vi "Mode Scan Engine.vi"() -> ()   [LabVIEW 2014]
uses:
  Controls/Standard Action.ctl
  Controls/Standard_Counter_Action.ctl
  <vilib>/Analysis/6fits.llb/Curve Fitting Criteria.ctl
  <vilib>/Analysis/baseanly.llb/Mean (DBL).vi
  <vilib>/Analysis/NI_AALBase.lvlib
  <vilib>/Analysis/NI_AALPro.lvlib
  <vilib>/gmath/NI_Gmath.lvlib
panel:
  in  "Initial Guess":T1={"Amp"=7.0, "Center"=7.0, "Sigma"=7.0, "Offset"=7.0}
  in  "Manual Initial Guess":bool
  in  "Upper Limit":dbl=7.0
  in  "Lower Limit":dbl=7.0
  out "Metric":cluster{dbl[], dbl[]}[](graph)
  out "Image":sgl[][](graph)
  in  "Step Size (nm)":u16=7
  in  "Number of Steps":u16=7
  in  "Get Image":bool
  in  "Scan Next Mode":bool
  in  "Metric":u16(ring) items=["Max Intensity", "No Zero Mean", "Threshold Mean"]
  in  "Fit Type":u16(ring) items=["Guassian", "Quadratic"]
  in  "Mode":i32(ring) items=["1", "2", "3", "4", "5", "6", "7", "8", "9", "10", "11", "12", "13", "14", "15", "16", "17", "18", "19", "20", "21", "22", "23", "24", "25", "26", "27", "28", "29", "30", "31", "32", "33", "34", "35", "36", "37", "38", "39", "40", "41", "42", "43", "44", "45", "46", "47", "48", "49", "50", "51", "52", "53", "54", "55", "56", "57", "58", "59", "60", "61", "62", "63", "64", "65", "66", "67", "68", "69", "70", "71", "72", "73", "74", "75", "76", "77", "78", "79", "80", "81", "82", "83", "84", "85", "86", "87", "88", "89", "90", "91", "92", "93", "94", "95", "96", "97", "98", "99", "100", "101", "102", "103", "104", "105", "106", "107", "108", "109", "110", "111", "112", "113", "114", "115", "116", "117", "118", "119", "120", "121", "122", "123", "124", "125", "126", "127", "128", "129", "130", "131", "132", "133", "134", "135", "136", "137", "138", "139", "140"]
  in  "Apply":bool
  in  "Fit Data":bool
  in  "Scan Mode":bool
  in  "Exit":bool
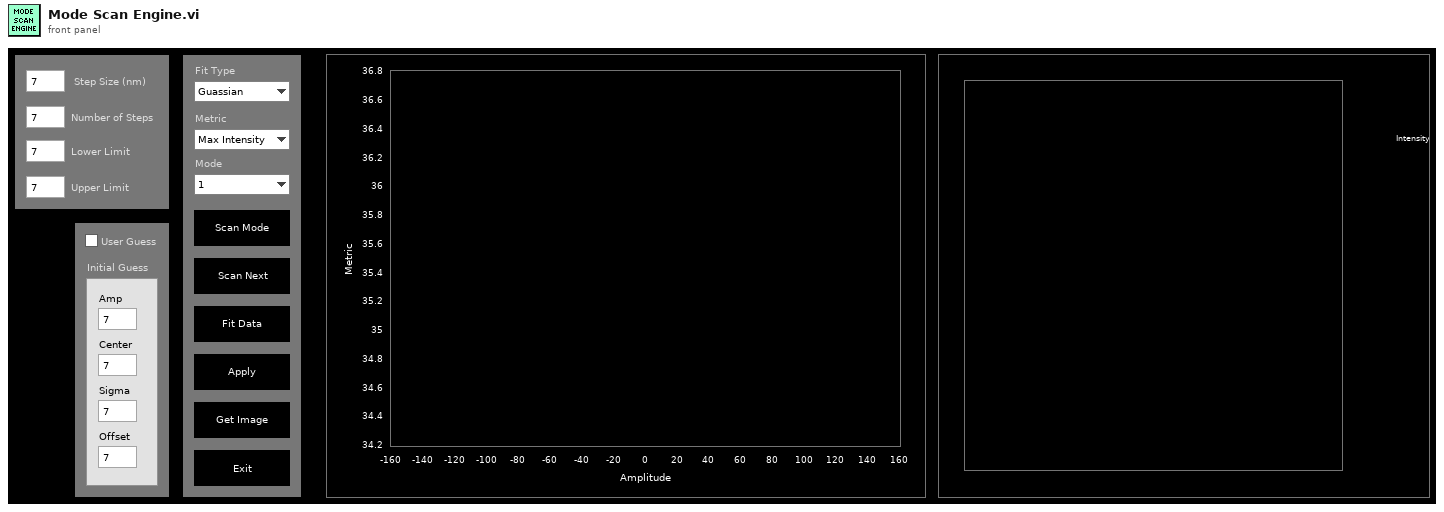
[diagram p1: front panel]
types:
  T1 = cluster{"Amp":dbl, "Center":dbl, "Sigma":dbl, "Offset":dbl}
  T2 = typedef "Standard Action.ctl" = enum16{"Read", "Write"}
  T3 = typedef "MirrorModes.ctl" = cluster{"Mode":string, "Amplitude":dbl}[]
  T4 = typedef "Standard_Counter_Action.ctl" = enum16{"Initialize", "Update Count", "Get Count"}
  T5 = cluster{"amp min":dbl, "amp max":dbl, "center min":dbl, "center max":dbl, "deviation min":dbl, "deviation max":dbl, "offset min":dbl, "offset max":dbl}
  T6 = enum16{"Linear", "Polynomial", "Exponential", "Power"}
  T7 = cluster{"Amplitude Out":dbl[], "Metric Out":dbl[]}
  T8 = cluster{"Amp":dbl, "Numeric":dbl, "Sigma":dbl, "Offset":dbl}
  T9 = typedef "NI_AALPro.lvlib/Curve Fitting Criteria.ctl" = u16
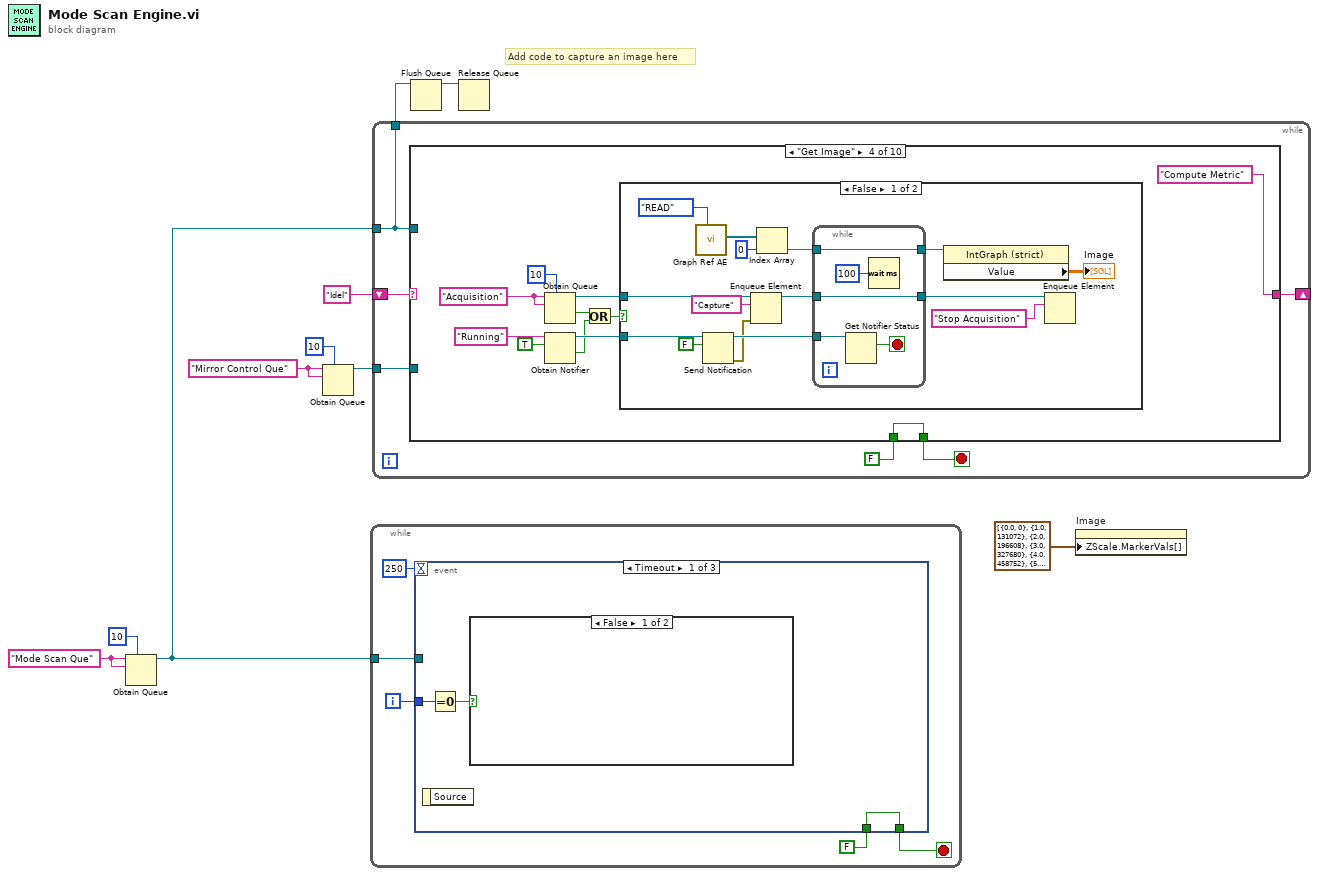
[diagram p0: block diagram]
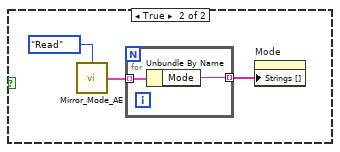
[diagram p2: hidden frame]
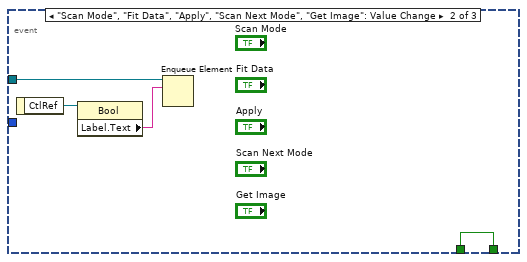
[diagram p3: hidden frame]
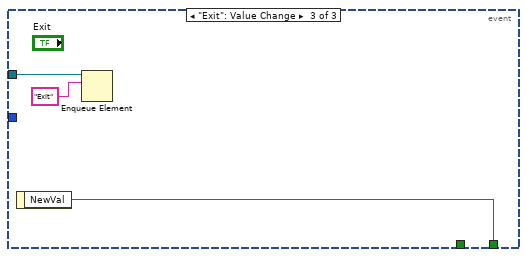
[diagram p4: hidden frame]
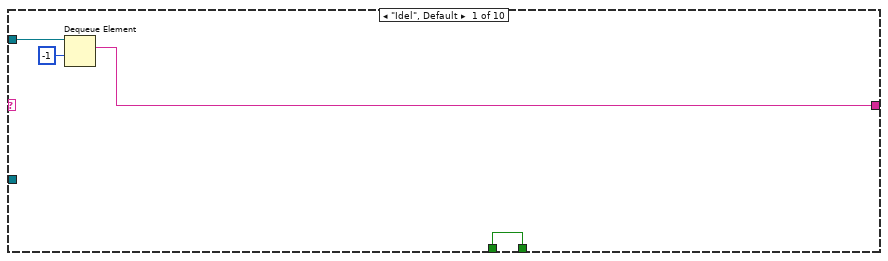
[diagram p5: hidden frame]
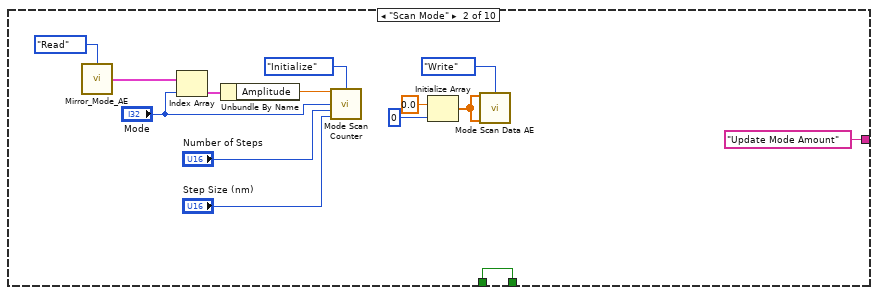
[diagram p6: hidden frame]
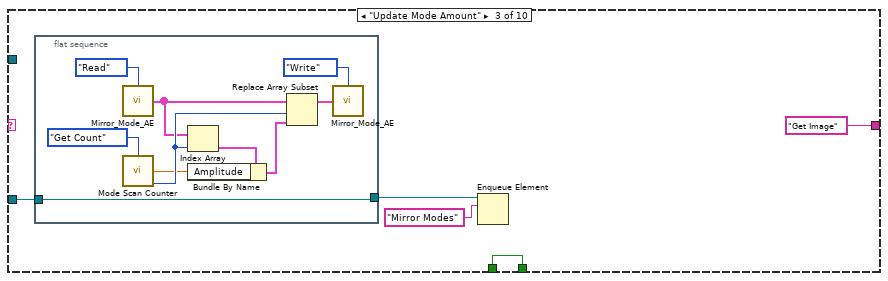
[diagram p7: hidden frame]
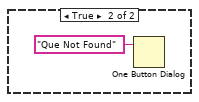
[diagram p8: hidden frame]
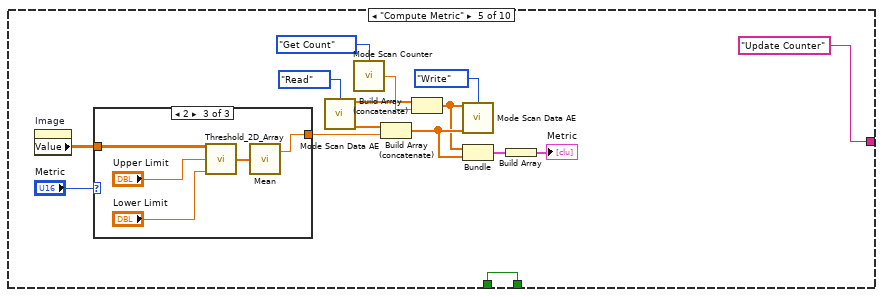
[diagram p9: hidden frame]
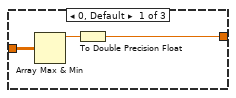
[diagram p10: hidden frame]
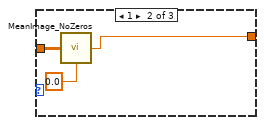
[diagram p11: hidden frame]
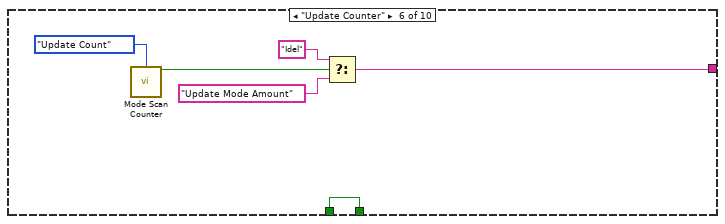
[diagram p12: hidden frame]
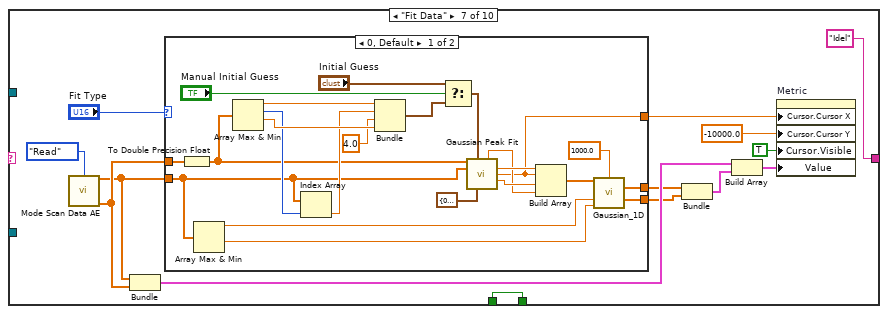
[diagram p13: hidden frame]
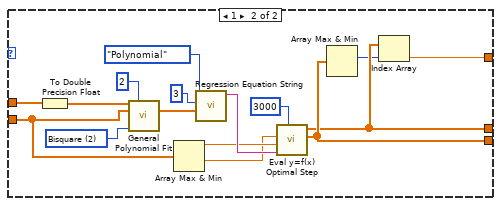
[diagram p14: hidden frame]
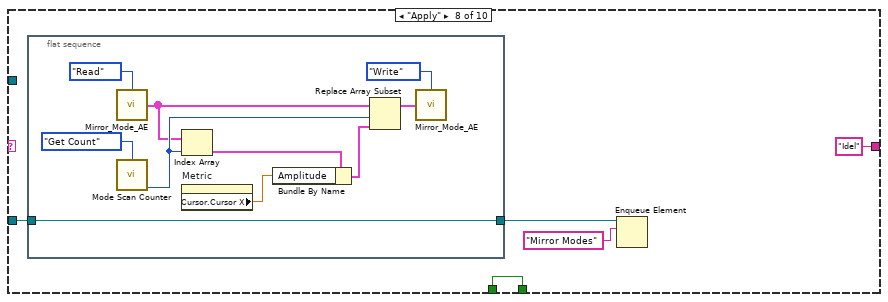
[diagram p15: hidden frame]
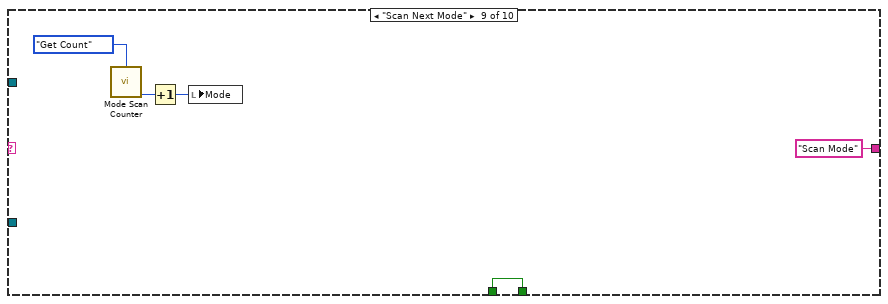
[diagram p16: hidden frame]
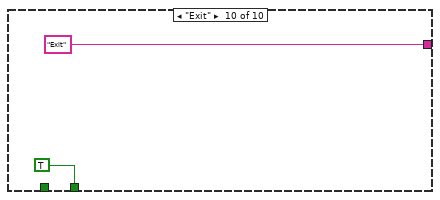
[diagram p17: hidden frame]
diagram:
  w4 = "Mirror Control Que" ("name (unnamed)")
  w9 = "Mode Scan Que" ("name (unnamed)")
  # "Add code to capture an image here"
  n1 = Obtain Queue(max queue size (-1, unlimited)=10, name (unnamed)=w9, element data type=w9) -> (queue out=w7:refnum<queue>)  [unwired: 2 in, 2 out]
  n2 = Obtain Queue(max queue size (-1, unlimited)=10, name (unnamed)=w4, element data type=w4) -> (queue out=w2:refnum<queue>)  [unwired: 2 in, 2 out]
  n3 = while {
    tunnel: w7 -> [w15]
    i -> [w12]
    stop <- w14 stop-if-true
    n4 = event shown="[0] Timeout" {
      selector: _ -> [_ _ _]
      dyn-events: _ -> [_ _ _]
      timeout: 250 -> [_ _ _]
      tunnel: w15 -> [_ w26 w30]
      tunnel: [w18 w24 w28] -> w14
      tunnel: FALSE -> [w18 w24 _]
      tunnel: w12 -> [w17 _ _]
      event Timeout {
        n5 = event-data() -> ()  [unwired: 1 in, 1 out]
        n6 = Equal To 0?(x=w17) -> (x = 0?=w16:bool)
        n7 = case shown="False" w16 {
          frame False {
          }
          frame True {
            n8 = call "Mirror_Mode_AE.vi"("Action"=Standard_Action."Read") -> ("Mirror Modes Out"=w20:T3)  [unwired: 14 in]
            n9 = for {
              tunnel: w20 -> [w23] mode=indexing
              tunnel: [w22] -> w21 mode=indexing
              n10 = Unbundle By Name(w23) -> ("Mode"=w22:string)
            }
            n11 = property on="Mode" class="Ring (strict)"("Strings []"=w21) -> ()  [unwired: 2 in, 2 out]
          }
        }
      }
      event "Scan Mode", "Fit Data", "Apply", "Scan Next Mode", "Get Image": Value Change {
        n12 = event-data() -> ("CtlRef"=w25:refnum<vi>)  [unwired: 1 in]
        n13 = property class="Bool"(reference=w25) -> ("Label.Text"=w27:string)  [unwired: 1 in, 2 out]
        n14 = Enqueue Element(queue=w26, element=w27) -> ()  [unwired: 2 in, 3 out]
      }
      event "Exit": Value Change {
        n15 = event-data() -> ("NewVal"=w28:bool)  [unwired: 1 in]
        n16 = Enqueue Element(queue=w30, element="Exit") -> ()  [unwired: 2 in, 3 out]
      }
    }
  }
  n17 = while {
    shift-right: [w33] -> _
    shift-left: "Idel" -> [w36]
    tunnel: w7 -> [w32]
    tunnel: [w32] -> w6
    tunnel: w2 -> [w31]
    stop <- w35 stop-if-true
    n18 = case shown="\"Get Image\"" w36 {
      tunnel: [w40 w54 w59 w80 w115 w133 w147 w191 w206 TRUE] -> w35
      tunnel: FALSE -> [w40 w54 w59 w80 w115 w133 w147 w191 w206 _]
      tunnel: w32 -> [w38 _ _ _ _ _ _ _ _ _]
      tunnel: [w37 "Update Mode Amount" ("name (unnamed)") "Get Image" ("name (unnamed)") "Compute Metric" ("name (unnamed)") "Update Counter" ("name (unnamed)") w130 "Idel" ("name (unnamed)") "Idel" ("name (unnamed)") "Scan Mode" ("name (unnamed)") "Exit" ("name (unnamed)")] -> w33
      tunnel: w31 -> [_ _ w58 _ _ _ _ w189 _ _]
      frame "Idel", Default {
        n19 = Dequeue Element(queue=w38, timeout in ms (-1)=-1) -> (element=w37:string)  [unwired: 1 in, 3 out]
      }
      frame "Scan Mode" {
        n20 = call "Mirror_Mode_AE.vi"("Action"=Standard_Action."Read") -> ("Mirror Modes Out"=w49:T3)  [unwired: 14 in]
        n21 = Index Array(array=w49, index="Mode") -> (element=w50:cluster{"Mode":string, "Amplitude":dbl})
        n22 = Unbundle By Name(w50) -> ("Amplitude"=w51:dbl)
        n23 = call "Mode Scan Counter.vi"("Center Value"=w51, "Action"=Standard_Counter_Action."Initialize", "Mode"="Mode", "Number of Steps"="Number of Steps", "Step Size"="Step Size (nm)") -> ()  [unwired: 8 in, 3 out]
        n24 = Initialize Array(0.0 ("element"), 0 ("dimension size")) -> (w41:dbl[])
        n25 = call "Mode Scan Data AE.vi"("Amplitude"=w41, "Action"=Standard_Action."Write", "Metric"=w41) -> ()  [unwired: 11 in, 2 out]
      }
      frame "Update Mode Amount" {
        n26 = flat-sequence {
          tunnel: w58 -> [w60]
          tunnel: [w60] -> w56
          frame #0 {
            n27 = call "Mirror_Mode_AE.vi"("Action"=Standard_Action."Read") -> ("Mirror Modes Out"=w63:T3)  [unwired: 14 in]
            n28 = call "Mode Scan Counter.vi"("Action"=Standard_Counter_Action."Get Count") -> ("Output"=w67:dbl, "Current Mode"=w68:i32)  [unwired: 12 in, 1 out]
            n29 = Index Array(array=w63, index=w68) -> (element=w66:cluster{"Mode":string, "Amplitude":dbl})
            n30 = Bundle By Name(cluster=w66, "Amplitude"=w67) -> (w69:cluster{"Mode":string, "Amplitude":dbl})
            n31 = Replace Array Subset(array=w63, new element=w69, index=w68) -> (w65:T3)
            n32 = call "Mirror_Mode_AE.vi"("Action"=Standard_Action."Write", "Mirror Modes In"=w65) -> ()  [unwired: 13 in, 1 out]
          }
        }
        n33 = Enqueue Element(queue=w56, element="Mirror Modes" ("name (unnamed)")) -> ()  [unwired: 2 in, 3 out]
      }
      frame "Get Image" {
        w75 = "Acquisition" ("name (unnamed)")
        n34 = Obtain Queue(max queue size (-1, unlimited)=10, name (unnamed)=w75, element data type=w75) -> (queue out=w78:refnum<queue>, created new?=w72:bool)  [unwired: 2 in, 1 out]
        n35 = Obtain Notifier(name (unnamed)="Running", notification data type=TRUE) -> (notifier out=w77:refnum<notifier>, created new?=w71:bool)  [unwired: 2 in, 1 out]
        n36 = Or(x=w72, y=w71) -> (x .or. y?=w70:bool)
        n37 = case shown="False" w70 {
          tunnel: w78 -> [w84 _]
          tunnel: w77 -> [w82 _]
          frame False {
            n38 = call "Graph Ref AE.vi"("Action"=enum16{"READ", "WRITE"}."READ") -> ("Graph Ref Out"=w92:refnum<vi>[])  [unwired: 10 in]
            n39 = Send Notification(notification=FALSE, notifier=w82) -> (notifier out=w87:refnum<notifier>, error out=w86:errorcluster)  [unwired: 1 in]
            n40 = Enqueue Element(queue=w84, element="Capture", error in (no error)=w86) -> (queue out=w88:refnum<queue>)  [unwired: 1 in, 2 out]
            n41 = Index Array(array=w92, index=0) -> (element=w94:refnum<vi>)
            n42 = while {
              tunnel: w87 -> [w100]
              tunnel: [w98] -> w89
              tunnel: w88 -> [w98]
              tunnel: [w97] -> w95
              tunnel: w94 -> [w97]
              stop <- w99 stop-if-true
              n43 = Get Notifier Status(notifier=w100) -> (current notification=w99:bool)  [unwired: 1 in, 4 out]
              n44 = Wait (ms)(milliseconds to wait=u32 100) -> ()  [unwired: 1 out]
            }
            n45 = property class="IntGraph (strict)"(reference=w95) -> ("Value"=→"Image":sgl[][])  [unwired: 1 in, 2 out]
            n46 = Enqueue Element(queue=w89, element="Stop Acquisition" ("f")) -> ()  [unwired: 2 in, 3 out]
          }
          frame True {
            n47 = One Button Dialog(message="Que Not Found") -> ()  [unwired: 1 in, 1 out]
          }
        }
      }
      frame "Compute Metric" {
        n48 = property on="Image" class="IntGraph (strict)"() -> ("Value"=w102:sgl[][])  [unwired: 2 in, 2 out]
        n49 = case shown="2" "Metric" {
          tunnel: w102 -> [w119 w122 w127]
          tunnel: [w117 w121 w125] -> w109
          frame 0, Default {
            n50 = Array Max & Min(array=w119) -> (max value=w118:sgl)  [unwired: 3 out]
            n51 = To Double Precision Float(number=w118) -> (double precision float=w117:dbl)
          }
          frame 1 {
            n52 = call "MeanImage_NoZeros.vi"("Image IN"=w122, "STDev Factor"=0.0) -> ("No Zero Mean"=w121:dbl)  [unwired: 13 in]
          }
          frame 2 {
            n53 = call "Threshold_2D_Array.vi"("2D Array IN"=w127, "Upper Limit"="Upper Limit", "Lower Limit"="Lower Limit") -> ("Threshold Array Out"=w126:dbl[])  [unwired: 12 in]
            n54 = call-poly <vilib>:"Mean.vi"("X"=w126) -> ("mean"=w125:dbl)  [unwired: 1 out]
          }
        }
        n55 = call "Mode Scan Data AE.vi"("Action"=Standard_Action."Read") -> ("Amplitude Out"=w106:dbl[], "Metric Out"=w107:dbl[])  [unwired: 13 in]
        n56 = call "Mode Scan Counter.vi"("Action"=Standard_Counter_Action."Get Count") -> ("Output"=w108:dbl)  [unwired: 12 in, 2 out]
        n57 = Build Array (concatenate)(w107, w109) -> (w112:dbl[])
        n58 = Build Array (concatenate)(w106, w108) -> (w111:dbl[])
        n59 = call "Mode Scan Data AE.vi"("Amplitude"=w111, "Action"=Standard_Action."Write", "Metric"=w112) -> ()  [unwired: 11 in, 2 out]
        n60 = Bundle(w111, w112) -> (w113:cluster{dbl[], dbl[]})  [unwired: 1 in]
        n61 = Build Array(w113) -> (→"Metric":cluster{dbl[], dbl[]}[])
      }
      frame "Update Counter" {
        n62 = call "Mode Scan Counter.vi"("Action"=Standard_Counter_Action."Update Count") -> ("Scan Done?"=w128:bool)  [unwired: 12 in, 2 out]
        n63 = Select(t="Idel", s=w128, f="Update Mode Amount") -> (s? t:f=w130:string)
      }
      frame "Fit Data" {
        n64 = call "Mode Scan Data AE.vi"("Action"=Standard_Action."Read") -> ("Amplitude Out"=w142:dbl[], "Metric Out"=w143:dbl[])  [unwired: 13 in]
        n65 = Bundle("Amplitude Out"=w142, "Metric Out"=w143) -> (w141:T7)  [unwired: 1 in]
        n66 = case shown="0, Default" "Fit Type" {
          tunnel: w142 -> [w163 w176]
          tunnel: w143 -> [w170 w175]
          tunnel: [w151 w172] -> w136
          tunnel: [w150 w173] -> w139
          tunnel: [w149 w174] -> w138
          frame 0, Default {
            n67 = To Double Precision Float(number=w170) -> (double precision float=w164:dbl[])
            n68 = Array Max & Min(array=w163) -> (max value=w152:dbl, min value=w153:dbl)  [unwired: 2 out]
            n69 = Array Max & Min(array=w164) -> (max value=w169:dbl, max index (indices)=w166:i32, min value=w168:dbl)  [unwired: 1 out]
            n70 = Index Array(array=w163, index=w166) -> (element=w165:dbl)
            n71 = Bundle(w169, "Numeric"=w165, 4.0, w168) -> (w162:cluster{dbl, "Numeric":dbl, dbl, dbl})  [unwired: 1 in]
            n72 = Select(t="Initial Guess", s="Manual Initial Guess", f=w162) -> (s? t:f=w161:T8)
            n73 = call <vilib>:"Gaussian Peak Fit.vi"("Y"=w164, "initial guess"=w161, "X"=w163, "parameter bounds"=T5 {"amp min"=0.0, "amp max"=100000.0, "center min"=-100.0, "center max"=100.0, "deviation min"=0.0, "deviation max"=1000.0, "offset min"=0.0, "offset max"=1000.0}) -> ("offset"=w156:dbl, "amplitude"=w158:dbl, "center"=w151:dbl, "standard deviation"=w157:dbl)  [unwired: 5 in, 3 out]
            n74 = Build Array(w158, w151, w157, w156) -> (w155:dbl[])
            n75 = call "Gaussian_1D.vi"("Parameters In"=w155, "Number of Points"=1000.0, "Max X Value"=w152, "Min X Value"=w153) -> ("X Values"=w150:dbl[], "Y Values"=w149:dbl[])  [unwired: 10 in]
          }
          frame 1 {
            w185 = T9 2 items=["Least Square", "Least Absolute Residual", "Bisquare"] ("method")
            n76 = To Double Precision Float(number=w175) -> (double precision float=w186:dbl[])
            n77 = call <vilib>:"General Polynomial Fit.vi"("Y"=w186, "polynomial order"=2, "X"=w176, "method"=w185) -> ("Polynomial Coefficients"=w182:dbl[])  [unwired: 8 in, 3 out]
            n78 = Array Max & Min(array=w176) -> (max value=w178:dbl, min value=w177:dbl)  [unwired: 2 out]
            n79 = call "Regression Equation String.vi"("coefficients"=w182, "precision"=3, "fit type"=T6."Polynomial") -> ("Formula"=w180:string)  [unwired: 8 in]
            n80 = call <vilib>:"Eval y=f(x) Optimal Step.vi"("number of points"=u32 3000, "formula"=w180, "end"=w178, "start"=w177) -> ("Y Values"=w174:dbl[], "X Values"=w173:dbl[])  [unwired: 1 in, 2 out]
            n81 = Array Max & Min(array=w174) -> (max index (indices)=w171:i32)  [unwired: 3 out]
            n82 = Index Array(array=w173, index=w171) -> (element=w172:dbl)
          }
        }
        n83 = Bundle("X Values"=w139, "Y Values"=w138) -> (w137:cluster{"X Values":dbl[], "Y Values":dbl[]})  [unwired: 1 in]
        n84 = Build Array(w141, w137) -> (w140:cluster{"X Values":dbl[], "Y Values":dbl[]}[])
        n85 = property on="Metric" class="XYGraph (strict)"("Cursor.Cursor X"=w136, "Cursor.Cursor Y"=-10000.0 ("Cursor.Cursor Position:Cursor X"), "Cursor.Visible"=TRUE, "Value"=w140) -> ()  [unwired: 2 in, 2 out]
      }
      frame "Apply" {
        n86 = flat-sequence {
          tunnel: [w193] -> w187
          tunnel: w189 -> [w193]
          frame #0 {
            n87 = call "Mirror_Mode_AE.vi"("Action"=Standard_Action."Read") -> ("Mirror Modes Out"=w196:T3)  [unwired: 14 in]
            n88 = call "Mode Scan Counter.vi"("Action"=Standard_Counter_Action."Get Count") -> ("Current Mode"=w200:i32)  [unwired: 12 in, 2 out]
            n89 = Index Array(array=w196, index=w200) -> (element=w199:cluster{"Mode":string, "Amplitude":dbl})
            n90 = property on="Metric" class="XYGraph (strict)"() -> ("Cursor.Cursor X"=w192:dbl)  [unwired: 2 in, 2 out]
            n91 = Bundle By Name(cluster=w199, "Amplitude"=w192) -> (w201:cluster{"Mode":string, "Amplitude":dbl})
            n92 = Replace Array Subset(array=w196, new element=w201, index=w200) -> (w198:T3)
            n93 = call "Mirror_Mode_AE.vi"("Action"=Standard_Action."Write", "Mirror Modes In"=w198) -> ()  [unwired: 13 in, 1 out]
          }
        }
        n94 = Enqueue Element(queue=w187, element="Mirror Modes" ("name (unnamed)")) -> ()  [unwired: 2 in, 3 out]
      }
      frame "Scan Next Mode" {
        n95 = call "Mode Scan Counter.vi"("Action"=Standard_Counter_Action."Get Count") -> ("Current Mode"=w203:i32)  [unwired: 12 in, 2 out]
        n96 = Increment(x=w203) -> (x+1=w204:i32)
        n97 = local write "Mode"(w204) -> ()
      }
      frame "Exit" {
      }
    }
  }
  n98 = Flush Queue(queue=w6) -> (queue out=w5:refnum<queue>)  [unwired: 1 in, 2 out]
  n99 = Release Queue(queue=w5) -> ()  [unwired: 2 in, 3 out]
  n100 = property on="Image" class="IntGraph (strict)"("ZScale.MarkerVals[]"=cluster{dbl, u32}[] [{0.0, 0}, {1.0, 131072}, {2.0, 196608}, {3.0, 327680}, {4.0, 458752}, {5.0, 589824}, {6.0, 720896}, {7.0, 851971}, {8.0, 983043}, {9.0, 1114115}, {10.0, 1245187}, {11.0, 1376259}, {12.0, 1507331}, {13.0, 1638403}, {14.0, 1769475}, {15.0, 1769479}, {16.0, 2031623}, {17.0, 2162695}, {18.0, 2293767}, {19.0, 2424839}, {20.0, 2555911}, {21.0, 2686983}, {22.0, 2818055}, {23.0, 2949127}, {24.0, 3080203}, {25.0, 3211275}, {26.0, 3342347}, {27.0, 3473419}, {28.0, 3604491}, {29.0, 3735563}, {30.0, 3866635}, {31.0, 3867403}, {32.0, 4129547}, {33.0, 4260619}, {34.0, 4391691}, {35.0, 4522763}, {36.0, 4653839}, {37.0, 4784911}, {38.0, 4915983}, {39.0, 5178127}, {40.0, 5309199}, {41.0, 5440271}, {42.0, 5571343}, {43.0, 5702415}, {44.0, 5703439}, {45.0, 5965583}, {46.0, 6096655}, {47.0, 6227727}, {48.0, 6358799}, {49.0, 6489871}, {50.0, 6620943}, {51.0, 6752015}, {52.0, 6883087}, {53.0, 7015183}, {54.0, 7146255}, {55.0, 7277327}, {56.0, 7408399}, {57.0, 7539471}, {58.0, 7670543}, {59.0, 7801615}, {60.0, 8063759}, {61.0, 8194831}, {62.0, 8326927}, {63.0, 8457999}, {64.0, 8589075}, {65.0, 8720147}, {66.0, 8851219}, {67.0, 8982291}, {68.0, 9113363}, {69.0, 9114387}, {70.0, 9376531}, {71.0, 9507603}, {72.0, 9638675}, {73.0, 9769747}, {74.0, 9901843}, {75.0, 10032915}, {76.0, 10163987}, {77.0, 10229523}, {78.0, 10295059}, {79.0, 10427155}, {80.0, 10558227}, {81.0, 10689299}, {82.0, 10820371}, {83.0, 10886931}, {84.0, 10952467}, {85.0, 11083539}, {86.0, 11214611}, {87.0, 11215635}, {88.0, 11477779}, {89.0, 11543315}, {90.0, 11608851}, {91.0, 11740947}, {92.0, 11806483}, {93.0, 11872019}, {94.0, 12004115}, {95.0, 12135187}, {96.0, 12266259}, {97.0, 12267283}, {98.0, 12398355}, {99.0, 12529427}, {100.0, 12530451}, {101.0, 12595987}, {102.0, 12530451}, {103.0, 12793619}, {104.0, 12794131}, {105.0, 12794643}, {106.0, 13056787}, {107.0, 13057299}, {108.0, 13057811}, {109.0, 13188883}, {110.0, 13320979}, {111.0, 13386515}, {112.0, 13452563}, {113.0, 13584147}, {114.0, 13584659}, {115.0, 13585171}, {116.0, 13585683}, {117.0, 13717267}, {118.0, 13848339}, {119.0, 13849363}, {120.0, 13849875}, {121.0, 13850387}, {122.0, 13981459}, {123.0, 14113555}, {124.0, 14114067}, {125.0, 14114579}, {126.0, 14115091}, {127.0, 14246675}, {128.0, 14377747}, {129.0, 14378771}, {130.0, 14379283}, {131.0, 14379539}, {132.0, 14379795}, {133.0, 14380819}, {134.0, 14511891}, {135.0, 14643987}, {136.0, 14644503}, {137.0, 14645015}, {138.0, 14645527}, {139.0, 14646039}, {140.0, 14646551}, {141.0, 14778135}, {142.0, 14909207}, {143.0, 14910231}, {144.0, 14910747}, {145.0, 14911259}, {146.0, 14911771}, {147.0, 14912283}, {148.0, 14912797}, {149.0, 15044383}, {150.0, 15175455}, {151.0, 15175967}, {152.0, 15176479}, {153.0, 15176991}, {154.0, 15177507}, {155.0, 15178019}, {156.0, 15178531}, {157.0, 15310115}, {158.0, 15441701}, {159.0, 15441959}, {160.0, 15442215}, {161.0, 15442727}, {162.0, 15443243}, {163.0, 15443755}, {164.0, 15444269}, {165.0, 15444783}, {166.0, 15444783}, {167.0, 15576367}, {168.0, 15707953}, {169.0, 15708467}, {170.0, 15708979}, {171.0, 15708981}, {172.0, 15708983}, {173.0, 15710011}, {174.0, 15710523}, {175.0, 15711037}, {176.0, 15711039}, {177.0, 15711553}, {178.0, 15843139}, {179.0, 15974213}, {180.0, 15974215}, {181.0, 15974217}, {182.0, 15974219}, {183.0, 15975755}, {184.0, 15976271}, {185.0, 15976785}, {186.0, 15977299}, {187.0, 15977301}, {188.0, 15977815}, {189.0, 15978327}, {190.0, 15978331}, {191.0, 16109917}, {192.0, 16241503}, {193.0, 16241505}, {194.0, 16242019}, {195.0, 16242535}, {196.0, 16242537}, {197.0, 16242539}, {198.0, 16243563}, {199.0, 16243567}, {200.0, 16244081}, {201.0, 16244595}, {202.0, 16244599}, {203.0, 16244601}, {204.0, 16244603}, {205.0, 16245627}, {206.0, 16245631}, {207.0, 16245633}, {208.0, 16246147}, {209.0, 16246663}, {210.0, 16377735}, {211.0, 16508811}, {212.0, 16508815}, {213.0, 16509839}, {214.0, 16509843}, {215.0, 16509845}, {216.0, 16509847}, {217.0, 16510361}, {218.0, 16510875}, {219.0, 16510879}, {220.0, 16510881}, {221.0, 16510883}, {222.0, 16511399}, {223.0, 16511911}, {224.0, 16511915}, {225.0, 16511917}, {226.0, 16511919}, {227.0, 16511923}, {228.0, 16512437}, {229.0, 16512951}, {230.0, 16512955}, {231.0, 16512957}, {232.0, 16512959}, {233.0, 16512961}, {234.0, 16512963}, {235.0, 16512967}, {236.0, 16513481}, {237.0, 16513995}, {238.0, 16513999}, {239.0, 16514001}, {240.0, 16514003}, {241.0, 16514005}, {242.0, 16514007}, {243.0, 16514011}, {244.0, 16514013}, {245.0, 16514015}, {246.0, 16514019}, {247.0, 16514021}, {248.0, 16514023}, {249.0, 16514027}, {250.0, 16514029}, {251.0, 16514031}, {252.0, 16514035}, {253.0, 16514037}, {254.0, 16514039}, {255.0, 16514043}] ("Z Scale.Marker Values[]")) -> ()  [unwired: 2 in, 2 out]
